vi "Measure Current.vi"(8 "error in":errorcluster, 11 "Acopian in":refnum<class "Acopian.lvclass">) -> (0 "error out":errorcluster, 2 "Current":dbl, 3 "Acopian out":refnum<class "Acopian.lvclass">)   [LabVIEW 2019, in "Acopian.lvlib" / "Acopian.lvclass"]
uses:
  Library/Acopian.lvclass
  Library/Acopian.lvclass/Acopian.ctl
  Accessors/Read Local Resource.vi
  Accessors/Write Local Resource.vi
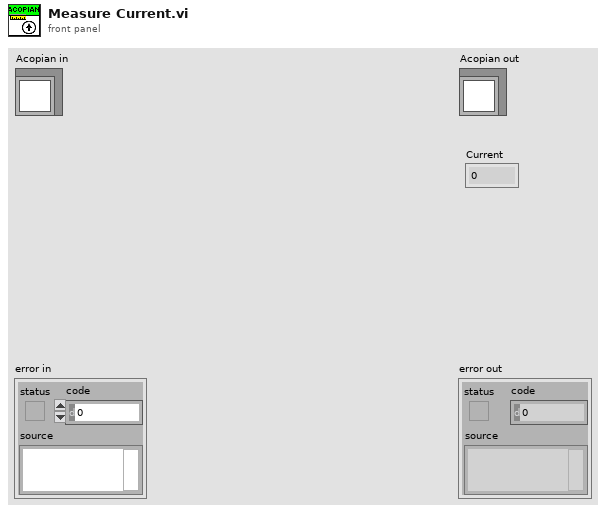
[diagram p1: front panel]
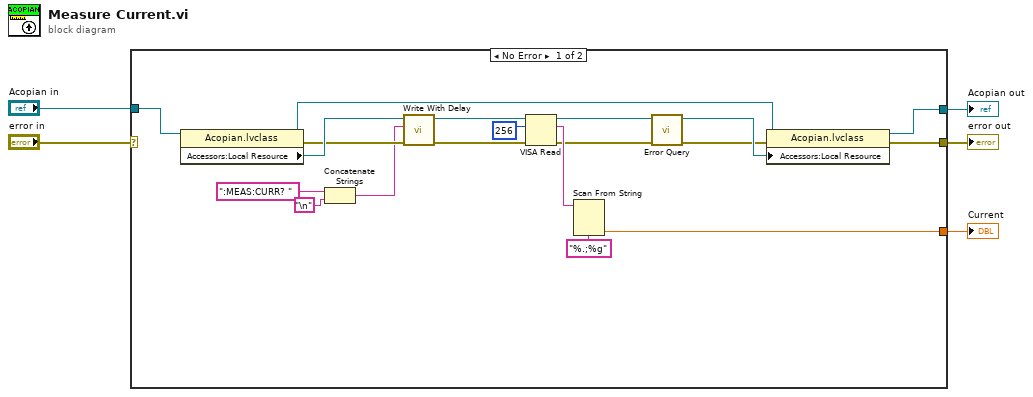
[diagram p0: block diagram]
diagram:
  n1 = case shown="No Error" "error in" {
    selector: "error in" -> [_ w26]
    tunnel: [w19 w26] -> w4
    tunnel: [w23 w25] -> w2
    tunnel: "Acopian in" -> [w24 w25]
    tunnel: [w6 _] -> w1
    frame No Error {
      n2 = property class="Acopian.lvclass"(reference=w24) -> (reference out=w22:refnum<class "Acopian.lvclass">, error out=w18:errorcluster, "Accessors:Local Resource"=w21:refnum<visa-resource-name>)  [unwired: 1 in]
      n3 = Concatenate Strings(":MEAS:CURR? " ("Current Measurement Command"), "\n") -> (w14:string)
      n4 = call "Write With Delay.vi"("error in"=w18, "write buffer"=w14, "VISA resource name"=w21) -> ("error out"=w11:errorcluster, "VISA resource name out"=w12:refnum<visa-resource-name>)  [unwired: 7 in]
      n5 = VISA Read(VISA resource name=w12, byte count=u32 256, error in (no error)=w11) -> (VISA resource name out=w9:refnum<visa-resource-name>, read buffer=w17:string, error out=w10:errorcluster)  [unwired: 1 out]
      n6 = Scan From String(format string="%.;%g", input string=w17) -> (output 1=w6:dbl)  [unwired: 3 in, 3 out]
      n7 = call "Error Query.vi"("error in"=w10, "VISA resource in"=w9) -> ("error out"=w7:errorcluster, "VISA resource out"=w8:refnum<visa-resource-name>)  [unwired: 6 in, 2 out]
      n8 = property class="Acopian.lvclass"(reference=w22, error in=w7, "Accessors:Local Resource"=w8) -> (reference out=w23:refnum<class "Acopian.lvclass">, error out=w19:errorcluster)
    }
    frame Error {
    }
  }
  "error out" <- w4
  "Acopian out" <- w2
  "Current" <- w1
